vi "svx_Waterfall Data at Constant Z.vi"(0 "cursors":T2[](array[typedef]), 1 "waterfall data":T1, 2 "z value (0)":dbl, 5 "error in (no error)":errorcluster) -> (14 "appended cursors":T2[](array[typedef]), 15 "duplicate waterfall data":T1, 16 "cursor data":cluster{"X":dbl, "Y":dbl, "Z":dbl}[](array[cluster]), 17 "cursor index":i32, 19 "error out":errorcluster)   [LabVIEW 2017]
doc: "Creates a cursor highlighting the data at a constant Z that can be plotted on a waterfall graph. Use the waterfall graph property node \"lines\" to draw the cursor on the graph."
uses:
  <vilib>/addons/_NISVFA/_Shared subVIs/Controls/svc_Cluster of Array of Cluster of XYZ.ctl
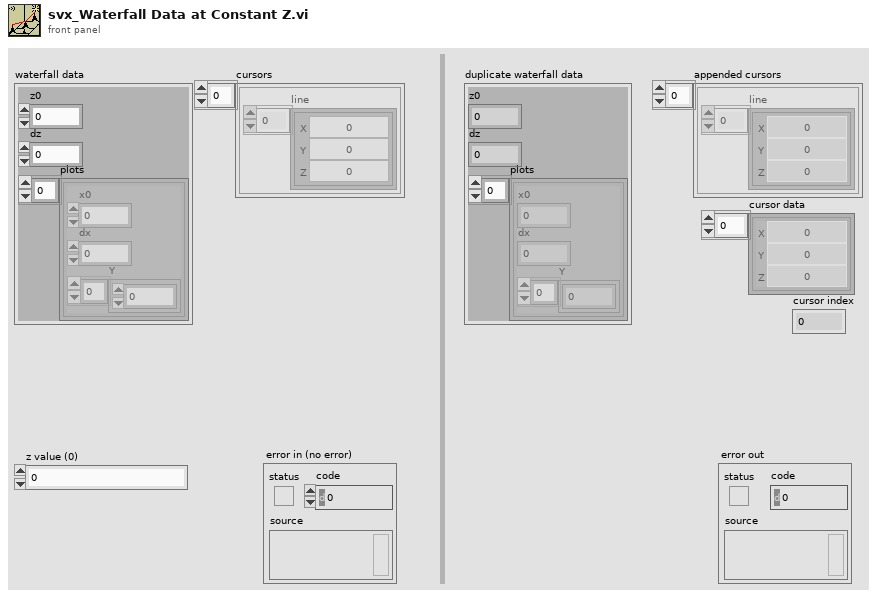
[diagram p1: front panel]
types:
  T1 = cluster{"z0":dbl, "dz":dbl, "plots":cluster{"x0":dbl, "dx":dbl, "Y":dbl[]}[]}
  T2 = typedef "svc_Cluster of Array of Cluster of XYZ.ctl" = cluster{"line":cluster{"X":dbl, "Y":dbl, "Z":dbl}[]}
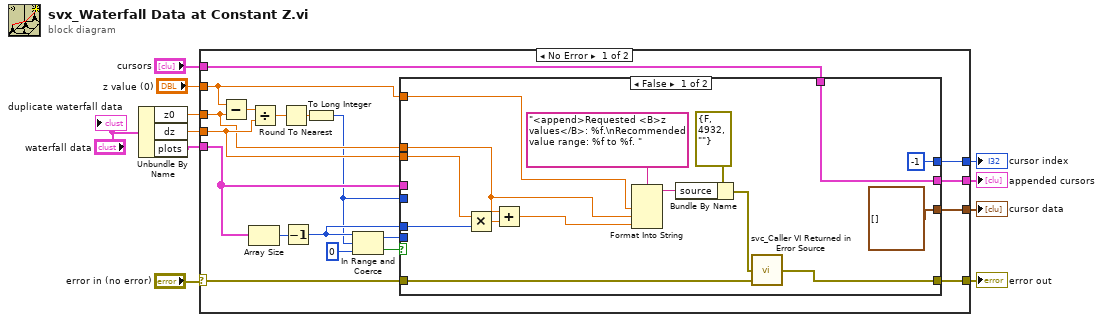
[diagram p0: block diagram]
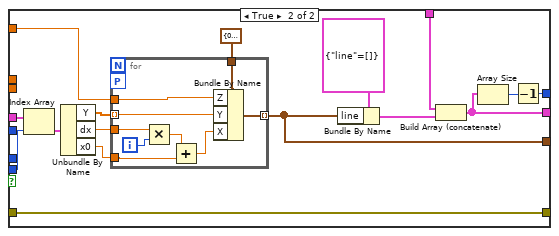
[diagram p2: hidden frame]
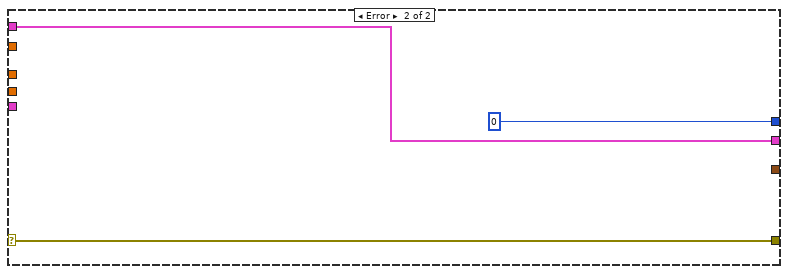
[diagram p3: hidden frame]
diagram:
  n1 = Unbundle By Name("waterfall data") -> ("z0"=w1:dbl, "dz"=w2:dbl, "plots"=w9:cluster{"x0":dbl, "dx":dbl, "Y":dbl[]}[])
  n2 = case shown="No Error" "error in (no error)" {
    selector: "error in (no error)" -> [w16 w73]
    tunnel: [w29 w72] -> w7
    tunnel: "z value (0)" -> [w12 _]
    tunnel: w9 -> [w20 _]
    tunnel: [w21 w73] -> w10
    tunnel: "cursors" -> [w30 w72]
    tunnel: [w22 _] -> w3
    tunnel: [w28 0] -> w4
    tunnel: w2 -> [w17 _]
    tunnel: w1 -> [w15 _]
    frame No Error {
      n3 = Subtract(x=w12, y=w15) -> (x-y=w26:dbl)
      n4 = Array Size(array=w20) -> (size(s)=w24:i32)
      n5 = Divide(x=w26, y=w17) -> (x/y=w27:dbl)
      n6 = Round To Nearest(number=w27) -> (nearest integer value=w25:dbl)
      n7 = Decrement(x=w24) -> (x-1=w18:i32)
      n8 = To Long Integer(number=w25) -> (32bit integer=w13:i32)
      n9 = In Range and Coerce(upper limit=w18, x=w13, lower limit=0) -> (coerced(x)=w19:i32, In Range?=w23:bool)
      n10 = case shown="False" w23 {
        tunnel: w30 -> [w44 w60]
        tunnel: [w44 w58] -> w29
        tunnel: [-1 w56] -> w28
        tunnel: [cluster{"X":dbl, "Y":dbl, "Z":dbl}[] [] w51] -> w22
        tunnel: [w35 w47] -> w21
        tunnel: w20 -> [_ w50]
        tunnel: w19 -> [_ w48]
        tunnel: w18 -> [w38 _]
        tunnel: w15 -> [w32 _]
        tunnel: w17 -> [w37 _]
        tunnel: w16 -> [w34 w47]
        tunnel: w13 -> [_ _]
        tunnel: w12 -> [w31 w46]
        frame False {
          n11 = Multiply(x=w37, y=w38) -> (x*y=w39:dbl)
          n12 = Add(x=w32, y=w39) -> (x+y=w33:dbl)
          n13 = Format Into String(format string="<append>Requested <B>z values</B>: %f.\nRecommended value range: %f to %f. ", w31, w32, w33) -> (resulting string=w40:string)  [unwired: 2 in, 1 out]
          n14 = Bundle By Name(cluster=errorcluster {"status"=FALSE, "code"=4932, "source"=""} ("error in (no error)"), "source"=w40) -> (w36:errorcluster)
          n15 = call <vilib>:"svc_Caller VI Returned in Error Source.vi"("warning input to caller"=w34, "error in (no error)"=w36) -> ("error out"=w35:errorcluster)  [unwired: 3 in]
        }
        frame True {
          n16 = Index Array(array=w50, index=w48) -> (element=w52:cluster{"x0":dbl, "dx":dbl, "Y":dbl[]})
          n17 = Unbundle By Name(w52) -> ("Y"=w54:dbl[], "dx"=w53:dbl, "x0"=w49:dbl)
          n18 = for {
            tunnel: cluster{"X":dbl, "Y":dbl, "Z":dbl} {"X"=0.0, "Y"=0.0, "Z"=0.0} -> [w70]
            tunnel: [w69] -> w51 mode=indexing
            workers-P: _ -> [_]
            tunnel: w54 -> [w68] mode=indexing
            tunnel: w53 -> [w66]
            tunnel: w46 -> [w65]
            tunnel: w49 -> [w62]
            i -> [w67]
            n19 = Multiply(x=w66, y=w67) -> (x*y=w64:dbl)
            n20 = Add(x=w64, y=w62) -> (x+y=w63:dbl)
            n21 = Bundle By Name(cluster=w70, "Z"=w65, "Y"=w68, "X"=w63) -> (w69:cluster{"X":dbl, "Y":dbl, "Z":dbl})
          }
          n22 = Bundle By Name(cluster=T2 {"line"=[]}, "line"=w51) -> (w59:T2)
          n23 = Build Array (concatenate)(w60, w59) -> (w58:T2[])
          n24 = Array Size(array=w58) -> (size(s)=w57:i32)
          n25 = Decrement(x=w57) -> (x-1=w56:i32)
        }
      }
    }
    frame Error {
    }
  }
  "error out" <- w10
  "appended cursors" <- w7
  "cursor index" <- w4
  "cursor data" <- w3
  "duplicate waterfall data" <- "waterfall data"
